vi "Update-sequence.vi"(8 "error in (no error)":errorcluster, 10 "Sequence":refnum<class "Action-sequence.lvclass">, 11 "Motor in":refnum<class "Motor.lvclass">) -> (0 "error out":errorcluster, 3 "Motor out":refnum<class "Motor.lvclass">)   [LabVIEW 2013, in "PowderDeposition.lvlib" / "Motor.lvclass"]
uses:
  Motor.lvclass
  Sequence/Action-sequence.lvclass
  Motor.lvclass/Motor.ctl
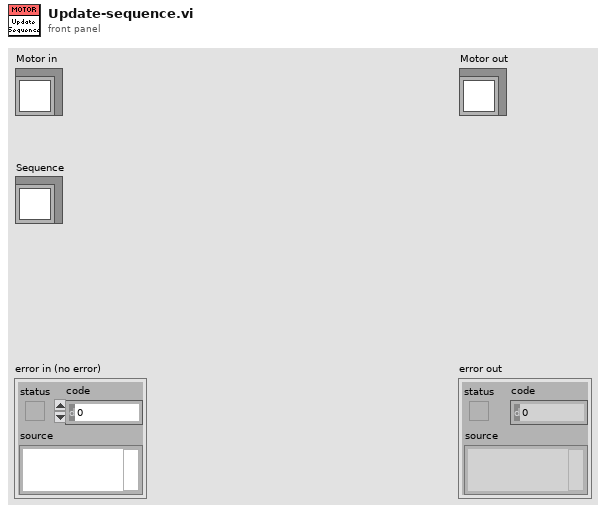
[diagram p1: front panel]
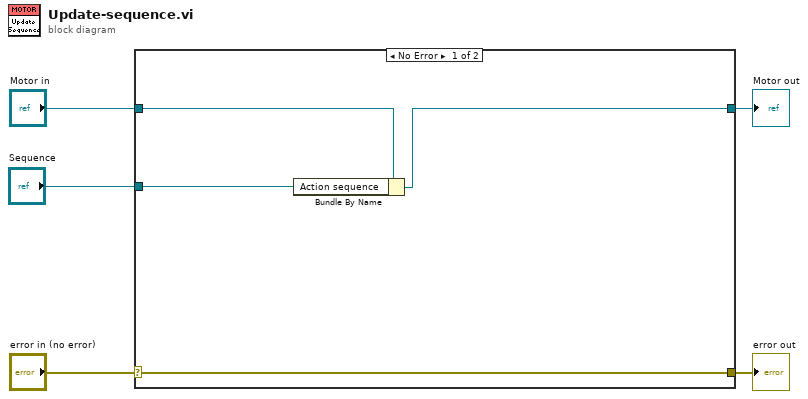
[diagram p0: block diagram]
diagram:
  n1 = case shown="No Error" "error in (no error)" {
    selector: "error in (no error)" -> [w9 w11]
    tunnel: [w9 w11] -> w4
    tunnel: [w6 w10] -> w2
    tunnel: "Motor in" -> [w7 w10]
    tunnel: "Sequence" -> [w8 _]
    frame No Error {
      n2 = Bundle By Name(cluster=w7, "Action sequence"=w8) -> (w6:refnum<class "Motor.lvclass">)
    }
    frame Error {
    }
  }
  "error out" <- w4
  "Motor out" <- w2
